vi "A_1.vi"() -> ()   [LabVIEW 2020]
panel:
  out "LED":bool
  in  "Dyscrimination level":dbl
  in  "Stop":bool
  out "Waveform Chart":cluster{"Dyscrimination level":dbl, dbl}(graph)
  in  "Noise amplitude":dbl
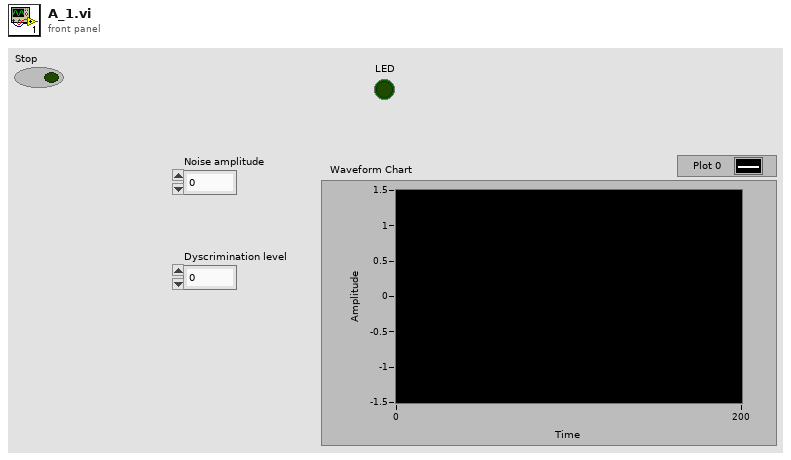
[diagram p1: front panel]
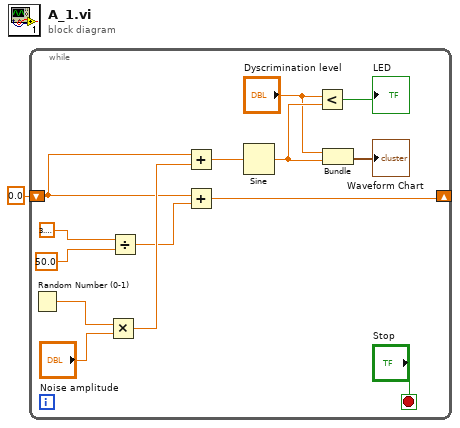
[diagram p0: block diagram]
diagram:
  n1 = while {
    shift-right: [w15] -> _
    shift-left: 0.0 -> [w11]
    stop <- "Stop" stop-if-true
    n2 = Random Number (0-1)() -> (number: 0 to 1=w14:dbl)
    n3 = Multiply(x=w14, y="Noise amplitude") -> (x*y=w12:dbl)
    n4 = Divide(x=3.141592653589793, y=50.0 ("x")) -> (x/y=w8:dbl)
    n5 = Add(x=w11, y=w12) -> (x+y=w10:dbl)
    n6 = Add(x=w11, y=w8) -> (x+y=w15:dbl)
    n7 = Sine(x=w10) -> (sin(x)=w3:dbl)
    n8 = Less?(x="Dyscrimination level", y=w3) -> (x < y?=→"LED":bool)
    n9 = Bundle("Dyscrimination level"="Dyscrimination level", w3) -> (→"Waveform Chart":cluster{"Dyscrimination level":dbl, dbl})  [unwired: 1 in]
  }
